vi "Configure Sweep (Ramp).vi"(0 "VISA resource name":refnum<visa-resource-name>, 1 "Enable Automatic Sweep Time (T:Enable)":bool=TRUE, 2 "Sweep Control Type (0: Master)":u16(ring) items=["Master", "Slave"], 3 "Sweep Control State (F:Disable)":bool, 5 "Sweep Time (10 ms)":dbl=0.01, 7 "Frequency Start (100 kHz)":dbl=100000.0, 9 "Frequency Stop (100 kHz)":dbl=100000.0, 11 "error in (no error)":errorcluster, 12 "Power Start (-135 dB)":dbl=-135.0, 13 "Power Stop (-135 dB)":dbl=-135.0) -> (4 "VISA resource name out":refnum<visa-resource-name>, 15 "error out":errorcluster)   [LabVIEW 2011, in "Agilent PSG MXG Series.lvlib"]
doc: "Configures sweep control, sweep time, start frequency, stop frequency, start amplitude and stop amplitude in the ramp sweep mode.\n\n<B>Notes:</B>\n(1) This VI is valid only in E8247C, E8257C, E8267C, E8257D, E8267D that install <B>Option 007</B> (Analog ramp sweep)."
uses:
  Agilent PSG MXG Series.lvlib
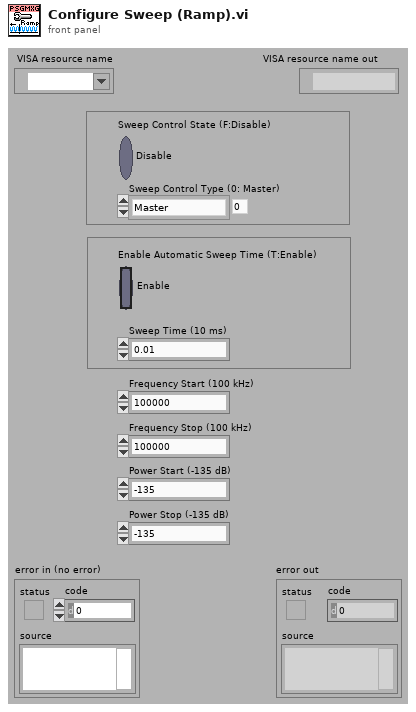
[diagram p1: front panel]
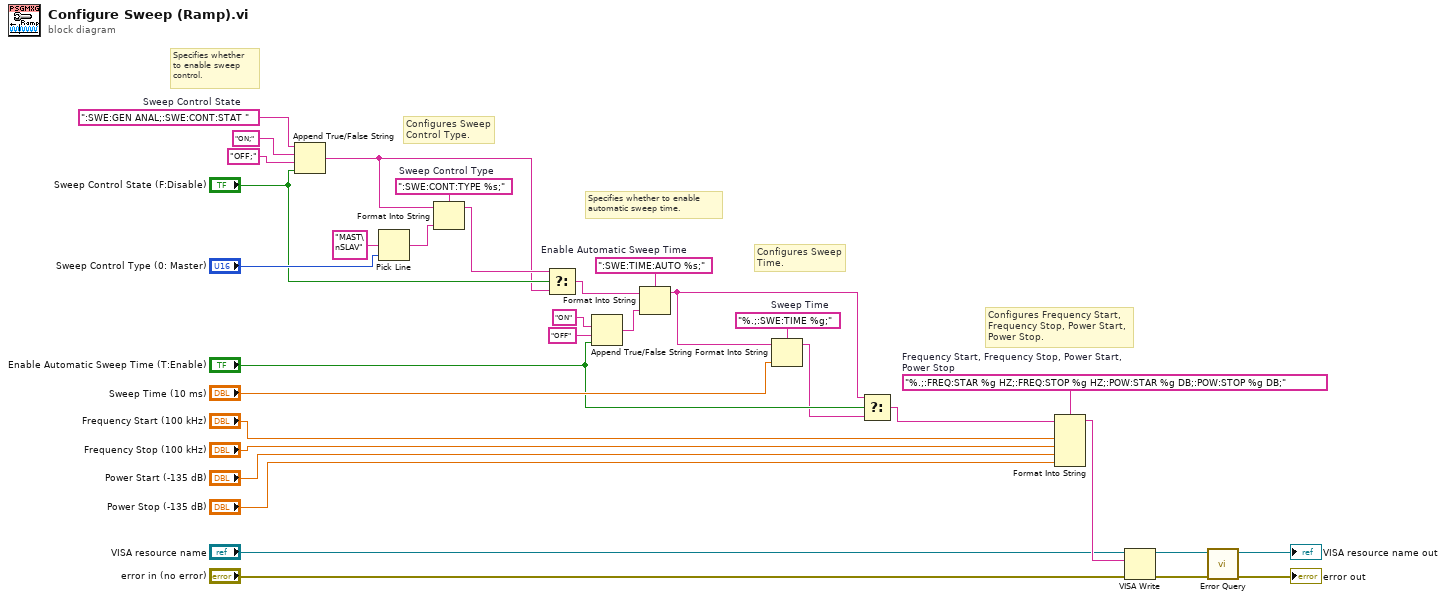
[diagram p0: block diagram]
diagram:
  w12 = "%.;:FREQ:STAR %g HZ;:FREQ:STOP %g HZ;:POW:STAR %g DB;:POW:STOP %g DB;"  # Frequency Start, Frequency Stop, Power Start, Power Stop
  w18 = "%.;:SWE:TIME %g;"  # Sweep Time
  w22 = ":SWE:TIME:AUTO %s;"  # Enable Automatic Sweep Time
  w30 = ":SWE:CONT:TYPE %s;"  # Sweep Control Type
  w33 = ":SWE:GEN ANAL;:SWE:CONT:STAT "  # Sweep Control State
  # "Configures Frequency Start,\nFrequency Stop, Power Start,\nPower Stop."
  # "Configures Sweep\nTime."
  # "Specifies whether to enable\nautomatic sweep time."
  # "Configures Sweep\nControl Type."
  # "Specifies whether\nto enable sweep\ncontrol."
  n1 = Append True/False String(1:"Sweep Control State (F:Disable)", 2:"OFF;" ("false string"), 3:"ON;" ("true string"), 4:w33) -> (0:w24:string)
  n2 = Pick Line(multi-line string="MAST\nSLAV", line index="Sweep Control Type (0: Master)") -> (output string=w29:string)  [unwired: 1 in]
  n3 = Format Into String(format string=w30, initial string=w24, w29) -> (resulting string=w25:string)  [unwired: 1 in, 1 out]
  n4 = Select(t=w25, s="Sweep Control State (F:Disable)", f=w24) -> (s? t:f=w23:string)
  n5 = Append True/False String(1:"Enable Automatic Sweep Time (T:Enable)", 2:"OFF" ("false string"), 3:"ON" ("true string")) -> (0:w21:string)  [unwired: 1 in]
  n6 = Format Into String(format string=w22, initial string=w23, w21) -> (resulting string=w15:string)  [unwired: 1 in, 1 out]
  n7 = Format Into String(format string=w18, initial string=w15, "Sweep Time (10 ms)") -> (resulting string=w14:string)  [unwired: 1 in, 1 out]
  n8 = Select(t=w15, s="Enable Automatic Sweep Time (T:Enable)", f=w14) -> (s? t:f=w13:string)
  n9 = Format Into String(format string=w12, initial string=w13, "Frequency Start (100 kHz)", "Frequency Stop (100 kHz)", "Power Start (-135 dB)", "Power Stop (-135 dB)") -> (resulting string=w7:string)  [unwired: 1 in, 1 out]
  n10 = VISA Write(VISA resource name="VISA resource name", write buffer=w7, error in (no error)="error in (no error)") -> (VISA resource name out=w6:refnum<visa-resource-name>, error out=w5:errorcluster)  [unwired: 1 out]
  n11 = call "Error Query.vi"("error in (no error)"=w5, "VISA resource name"=w6) -> ("error out"=→"error out":errorcluster, "VISA resource name out"=→"VISA resource name out":refnum<visa-resource-name>)  [unwired: 6 in, 2 out]
